vi "myRIO_BRig_RT_dataLC_Selection_Block_Switch_l2.vi"() -> (2 "output_Selection_Block_Switch_l2":i32)   [LabVIEW 2014]
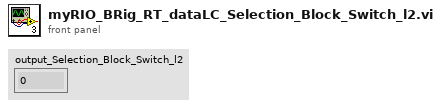
[diagram p1: front panel]
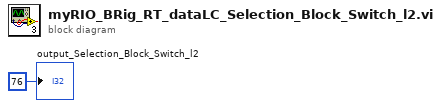
[diagram p0: block diagram]
diagram:
  "output_Selection_Block_Switch_l2" <- 76 ("output_iBlock")
